vi "Number Check.vi"(9 "string in":string) -> (4 "Number?":bool, 5 "String out":string)   [LabVIEW 2015, in "Touch_keyboard.lvlib"]
doc: "Name: Number Check\nAuthor:Georges Janveau, Columbia Forest Products\nCreated: 6/10/05\n\nDESCRIPTION\nVerifies the input string is a number\n\nINPUTS\n\nString In - The String to be verified.\n\nOUTPUTS\nString Out - Result (will contain String In if the String In is a number).\nNumber ?- Verification Result (T/F)\n\n----------------------------------------------------------------------------------------------------------------"
uses:
  Touch_keyboard.lvlib
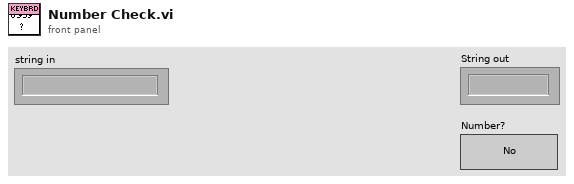
[diagram p1: front panel]
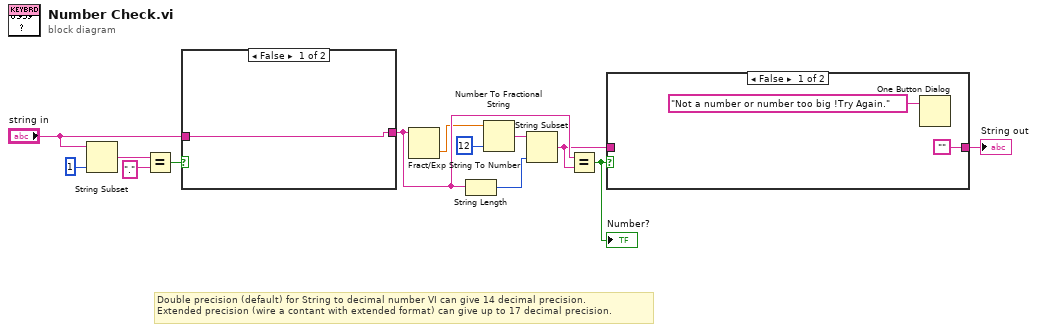
[diagram p0: block diagram]
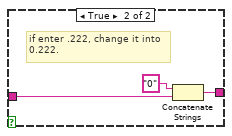
[diagram p3: hidden frame]
diagram:
  # "Double precision (default) for String to decimal number VI can give 14 decimal precision.\nExtended precision (wire a contant with extended format) can give up to 17 decimal precision."
  n1 = String Subset(string="string in", length (rest)=1 ("length")) -> (substring=w11:string)  [unwired: 1 in]
  n2 = Equal?(x=w11, y=".") -> (x = y?=w9:bool)
  n3 = case shown="False" w9 {
    tunnel: [w14 w15] -> w5
    tunnel: "string in" -> [w14 w16]
    frame False {
    }
    frame True {
      # "if enter .222, change it into\n0.222."
      n4 = Concatenate Strings("0", w16) -> (w15:string)
    }
  }
  n5 = Fract/Exp String To Number(string=w5) -> (number=w4:dbl)  [unwired: 3 in, 1 out]
  n6 = String Length(string=w5) -> (length=w3:i32)
  n7 = Number To Fractional String(number=w4, precision (6)=i16 12) -> (F-format string=w13:string)  [unwired: 2 in]
  n8 = String Subset(string=w13, length (rest)=w3) -> (substring=w2:string)  [unwired: 1 in]
  n9 = Equal?(x=w5, y=w2) -> (x = y?=w7:bool)
  "Number?" <- w7
  n10 = case shown="False" w7 {
    tunnel: w2 -> [_ w20]
    tunnel: ["" w20] -> w1
    frame False {
      n11 = One Button Dialog(message="Not a number or number too big !Try Again.") -> ()  [unwired: 1 in, 1 out]
    }
    frame True {
    }
  }
  "String out" <- w1
